vi "Send Open Front Panel.vi"(6 "Custom Window Size":cluster{"Height":i16, "Width":i16}={"Height"=-1, "Width"=-1}, 7 "Message Priority (Normal)":T2=enum."Normal", 8 "error in (no error)":errorcluster, 9 "Custom Window Position":cluster{"Top":i16, "Left":i16}={"Top"=-1, "Left"=-1}, 10 "Position":T1, 11 "Message Enqueuer":refnum<class "Message Enqueuer.lvclass">) -> (0 "error out":errorcluster, 3 "Message Enqueuer out":refnum<class "Message Enqueuer.lvclass">)   [LabVIEW 2017, in "IViewable.lvlib" / "Open Front Panel Msg.lvclass"]
doc: "This VI sends the message to an actor.\n\n<License>\nCopyright © 2017 Composed Systems, LLC | All rights reserved\nwww.composed.io\n\nAuthor: Ethan Stern <ethan.stern@composed.io>\n\nThis software is provided \"AS IS\" WITHOUT WARRANTIES, either express or implied, AND IS FOR EDUCATIONAL PURPOSES ONLY.\n</License>"
uses:
  Open Front Panel Msg.lvclass
  <vilib>/ActorFramework/Message Enqueuer/Message Enqueuer.lvclass
  <vilib>/ActorFramework/Message Enqueuer/Message Priority.ctl
  IViewable/View Position Enum.ctl
  C:/Program Files (x86)/National Instruments/LabVIEW 2017/vi.lib/ActorFramework/Message/Message.lvclass
  Open Front Panel Msg.lvclass/Open Front Panel Msg.ctl
  <vilib>/ActorFramework/Message Enqueuer/Message Enqueuer.lvclass/Message Enqueuer.ctl
  <vilib>/ActorFramework/Message Priority Queue/Priority Enqueue.vi
  IViewable/IViewable.lvclass
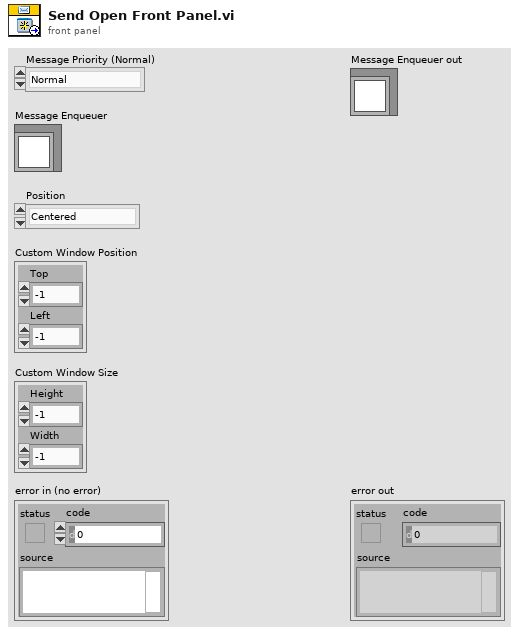
[diagram p1: front panel]
types:
  T1 = typedef "IViewable.lvlib/IViewable.lvclass/View Position Enum.ctl" = enum16{"Centered", "Maximized", "Minimized", "Custom", "Unchanged"}
  T2 = typedef "Actor Framework.lvlib/Message Enqueuer.lvclass/Message Priority.ctl" = enum16{"Low", "Normal", "High"}
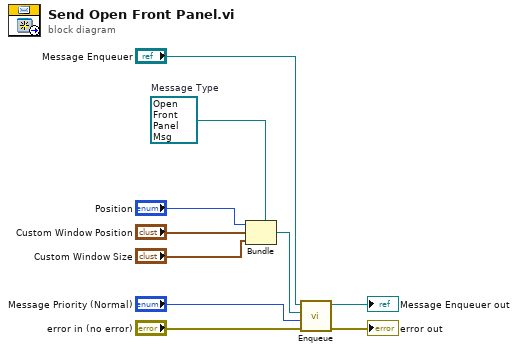
[diagram p0: block diagram]
diagram:
  w7 = refnum<class "Open Front Panel Msg.lvclass"> refnum  # Message Type
  n1 = Bundle(cluster=w7, "Position", "Custom Window Position", "Custom Window Size") -> (w6:refnum<class "Open Front Panel Msg.lvclass">)
  n2 = call <vilib>:"Enqueue.vi"("error in (no error)"="error in (no error)", "Message Priority (Normal)"="Message Priority (Normal)", "Message"=w6, "Message Enqueuer in"="Message Enqueuer") -> ("error out"=→"error out":errorcluster, "Message Enqueuer out"=→"Message Enqueuer out":refnum<class "Message Enqueuer.lvclass">)  [unwired: 6 in]
